vi "find_surface_simple1.vi"(8 "error in (no error)":errorcluster, 10 "Filter Size":i32=30, 11 "Image In":T1) -> (0 "error out":errorcluster, 3 "surface depth":dbl format="%0.2f")   [LabVIEW 2016]
doc: "Estimates position of top surface of B-scan using convolution."
uses:
  <vilib>/vision/Image Controls.llb/IMAQ Image.ctl
  <vilib>/vision/NI_Vision_Development_Module.lvlib
  <vilib>/Analysis/NI_AALBase.lvlib
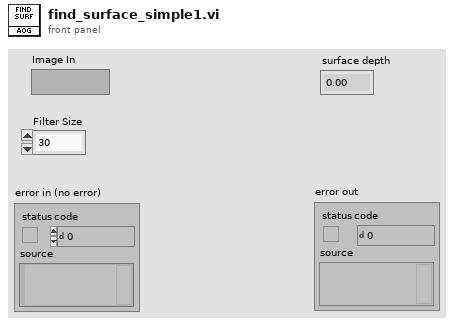
[diagram p1: front panel]
types:
  T1 = typedef "IMAQ Image.ctl" = refnum<image>
  T2 = typedef "Image Type" = u32
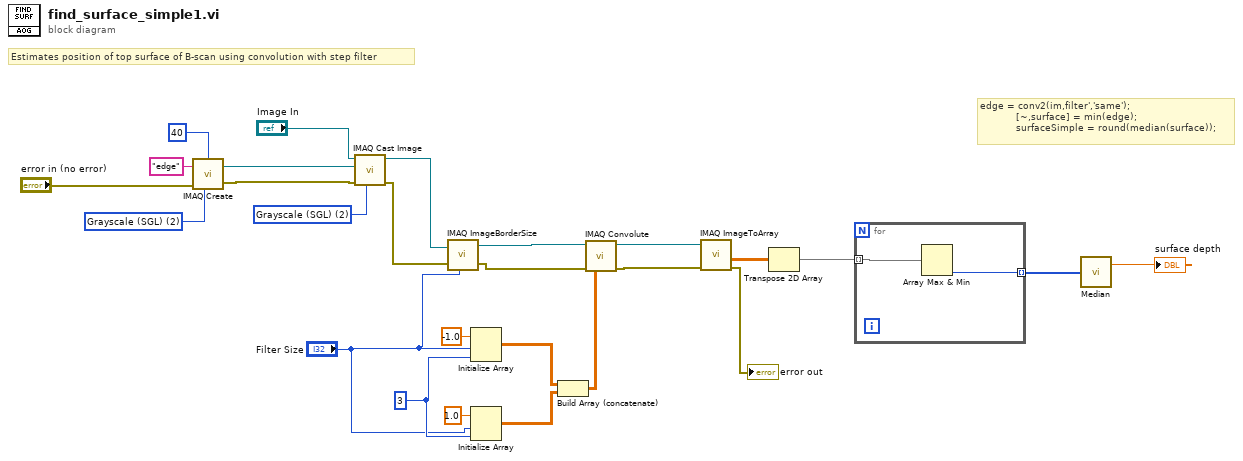
[diagram p0: block diagram]
diagram:
  w19 = 3 ("dimension size")
  w22 = T2 2 items=["Grayscale (U8)", "Grayscale (I16)", "Grayscale (SGL)", "Complex (CSG)", "RGB (U32)", "HSL (U32)", "RGB (U64)", "Grayscale (U16)"] ("Image Type")
  w25 = T2 2 items=["Grayscale (U8)", "Grayscale (I16)", "Grayscale (SGL)", "Complex (CSG)", "RGB (U32)", "HSL (U32)", "RGB (U64)", "Grayscale (U16)"] ("Image Type")
  # "Estimates position of top surface of B-scan using convolution with step filter"
  # "edge = conv2(im,filter','same');\n            [~,surface] = min(edge);\n            surfaceSimple = round(median(surface));"
  n1 = call "IMAQ Create"("Border Size"=40, "Image Name"="edge", "Image Type"=w25, "error in (no error)"="error in (no error)") -> ("New Image"=w24:T1, "error out"=w8:errorcluster)  [unwired: 1 in]
  n2 = call "IMAQ Cast Image"("Image Type"=w22, "error in (no error)"=w8, "Image Dst"=w24, "Image Src"="Image In") -> ("error out"=w7:errorcluster, "Image Dst Out"=w14:T1)  [unwired: 6 in]
  n3 = call "IMAQ ImageBorderSize"("Image"=w14, "Image border size in"="Filter Size", "error in (no error)"=w7) -> ("Image Out"=w13:T1, "error out"=w6:errorcluster)  [unwired: 1 in, 1 out]
  n4 = Initialize Array(-1.0 ("element"), "Filter Size", w19) -> (w18:dbl[][])
  n5 = Initialize Array(1.0 ("element"), "Filter Size", w19) -> (w17:dbl[][])
  n6 = Build Array (concatenate)(w18, w17) -> (w16:dbl[][])
  n7 = call "IMAQ Convolute"("Kernel"=w16, "error in (no error)"=w6, "Image Src"=w13) -> ("error out"=w5:errorcluster, "Image Dst Out"=w11:T1)  [unwired: 7 in]
  n8 = call "IMAQ ImageToArray"("error in (no error)"=w5, "Image"=w11) -> ("Image Pixels (Float)"=w3:sgl[][], "error out"=→"error out":errorcluster)  [unwired: 2 in, 3 out]
  n9 = Transpose 2D Array(2D array=w3) -> (transposed array=w2:sgl[][])
  n10 = for {
    tunnel: w2 -> [w28] mode=indexing
    tunnel: [w27] -> w1 mode=indexing
    n11 = Array Max & Min(array=w28) -> (min index (indices)=w27:i32)  [unwired: 3 out]
  }
  n12 = call <vilib>:"Median.vi"("X"=w1) -> ("median"=→"surface depth":dbl)  [unwired: 1 out]
